vi "Left Click.vi"(7 "object refs":T2, 8 "error in (no error)":errorcluster, 9 "Coords":T1, 10 "Event data":variant, 11 "Data Grid in":refnum<class "Data Grid.lvclass">) -> (0 "error out":errorcluster, 2 "Discard?":bool, 3 "Data Grid out":refnum<class "Data Grid.lvclass">)   [LabVIEW 2013, in "Table Manager.lvlib" / "Data Grid.lvclass"]
uses:
  Data Grid.lvclass
  Table Manager/object ref.ctl
  <vilib>/NI/Tag Bus Data Framework/Configuration Editor/Classes/Engine Parent/Engine Parent Editor Node.lvclass
  <vilib>/NI/Tag Bus Data Framework/Configuration Editor/Classes/Module editor node/module editor node.lvclass
  <vilib>/Utility/miscctls.llb/LVPoint32TypeDef.ctl
  <vilib>/LabVIEW DataGridView/source/Events/Abstract EVENT/Abstract EVENT.lvclass
  Data Grid.lvclass/Data Grid.ctl
  Table Manager/Table Manager.lvclass/Table Manager.ctl
  Line/Line.lvclass/Line.ctl
  Column/Column.lvclass/Column.ctl
  Column/Column.lvclass
  Table Manager/Read ATM.vi
  Table Manager/Read Line.vi
  Table Manager/Read Top VI.vi
  Line/Read Columns.vi
  Line/Write Columns.vi
  Table Manager/Write Line.vi
  <vilib>/NI/Tag Bus Data Framework/Configuration Editor/Classes/Module editor node/Read Module Configuration.vi
  Line/Line.lvclass
  <vilib>/NI/Tag Bus Module Framework/module configuration/TBM module configuration.lvclass
  <vilib>/LabVIEW DataGridView/source/Events/CellClick/CellClick.lvclass
  <vilib>/NI/Tag Bus/tag/tag descriptor.lvclass
  Table Manager.lvlib
  <vilib>/LabVIEW DataGridView/source/DataGridView/DataGridView.lvclass
  Table Manager/Table Manager.lvclass
  Mapping Column/Mapping Column.lvclass
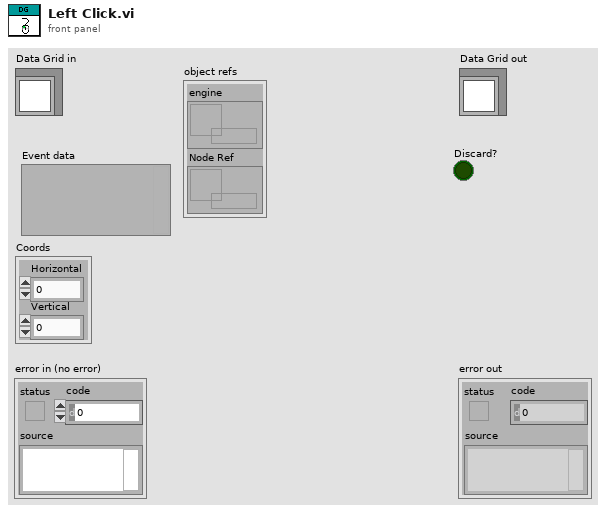
[diagram p1: front panel]
types:
  T1 = typedef "LVPoint32TypeDef.ctl" = cluster{"Horizontal":i32, "Vertical":i32}
  T2 = typedef "Table Manager.lvlib/Table Manager.lvclass/object ref.ctl" = cluster{"engine":refnum<data-value>, "Node Ref":refnum<data-value>}
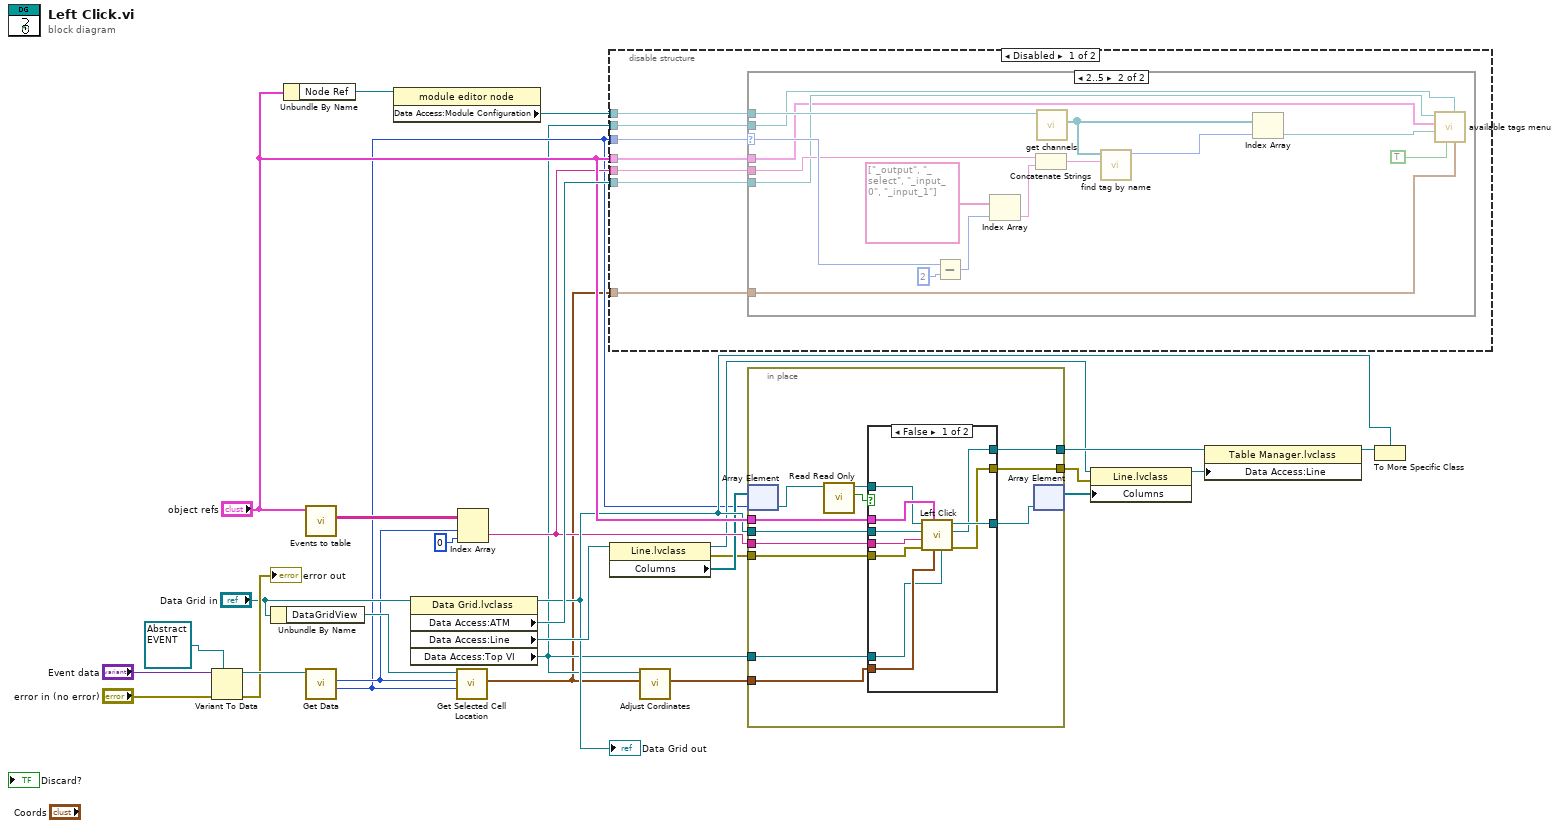
[diagram p0: block diagram]
diagram:
  n1 = Variant To Data(error in="error in (no error)", type=refnum<class "Abstract EVENT.lvclass"> refnum ("DataGrid.lvlib:Abstract EVENT.lvclass"), Variant="Event data") -> (data=w23:refnum<class "Abstract EVENT.lvclass">, error out=→"error out":errorcluster)
  n2 = Unbundle By Name("Data Grid in") -> ("DataGridView"=w22:refnum<class "DataGridView.lvclass">)
  n3 = Unbundle By Name("object refs") -> ("Node Ref"=w27:refnum<data-value>)
  n4 = call "Events to table.vi"("object ref in"="object refs") -> ("table"=w26:string[][])  [unwired: 8 in, 2 out]
  n5 = call <vilib>:"Get Data.vi"("DataGrid.lvlib:Abstract EVENT.lvclass"=w23) -> ("column"=w4:i32, "row"=w17:i32)  [unwired: 8 in, 1 out]
  n6 = property class="module editor node"(reference=w27) -> ("Data Access:Module Configuration"=w28:refnum<class "TBM module configuration.lvclass">)  [unwired: 1 in, 2 out]
  n7 = property class="Data Grid.lvclass"(reference="Data Grid in") -> (reference out=w14:refnum<class "Data Grid.lvclass">, "Data Access:ATM"=w18:refnum<user-event>, "Data Access:Line"=w16:refnum<class "Line.lvclass">, "Data Access:Top VI"=w3:refnum<vi>)  [unwired: 1 in, 1 out]
  "Data Grid out" <- w14
  n8 = call <vilib>:"Get Selected Cell Location.vi"("column"=w4, "row"=w17, "DataGridView in"=w22) -> ("Coords"=w2:T1)  [unwired: 7 in, 1 out]
  n9 = Index Array(array=w26, index (row)=w17, index (col)=0 ("disabled index (col)")) -> (element=w10:string)
  n10 = disable-structure shown="Disabled" {
    disable-tunnel: w2 -> [w36 _]
    disable-tunnel: w10 -> [w35 _]
    disable-tunnel: w28 -> [w34 _]
    disable-tunnel: w18 -> [w33 _]
    disable-tunnel: w4 -> [w32 _]
    disable-tunnel: w3 -> [w31 _]
    disable-tunnel: "object refs" -> [w30 _]
    frame Disabled {
      n11 = case shown="2..5" w32 {
        selector: w32 -> [_ w49]
        tunnel: w35 -> [_ w45]
        tunnel: w36 -> [_ w39]
        tunnel: w34 -> [_ w41]
        tunnel: w33 -> [_ w40]
        tunnel: w30 -> [_ w38]
        tunnel: w31 -> [_ w37]
        frame 0, Default {
        }
        frame 2..5 {
          n12 = Subtract(x=w49, y=2) -> (x-y=w48:i32)
          n13 = Index Array(array=string[] ["_output", "_select", "_input_0", "_input_1"], index=w48) -> (element=w44:string)
          n14 = Concatenate Strings(w45, w44) -> (w46:string)
          n15 = call-dynamic "get channels.vi"("module configuration in"=w41) -> ("channels"=w42:refnum<class "TBM channel.lvclass">[])  [unwired: 9 in, 1 out]
          n16 = call <vilib>:"find tag by name.vi"("name"=w46, "tags in"=w42) -> ("index"=w52:i32)  [unwired: 9 in]
          n17 = Index Array(array=w42, index=w52) -> (element=w51:refnum<class "TBM channel.lvclass">)
          n18 = call "available tags menu.vi"("Point32"=w39, "parent vi reference"=w37, "Screen"=TRUE, "channel to map to"=w51, "object ref"=w38, "ATM"=w40) -> ()  [unwired: 5 in, 1 out]
        }
      }
    }
    frame Enabled {
    }
  }
  n19 = property class="Line.lvclass"(reference=w16) -> (reference out=w7:refnum<class "Line.lvclass">, error out=w6:errorcluster, "Columns"=w9:refnum<class "Column.lvclass">[])  [unwired: 1 in]
  n20 = call "Adjust Cordinates.vi"("Point32"=w2, "VI in"=w3) -> ("Coords out"=w1:T1)  [unwired: 8 in, 1 out]
  n21 = in-place {
    in-place-border: "object refs" -> [w63]
    in-place-border: w14 -> [w62]
    in-place-border: [w61] -> w13
    in-place-border: w1 -> [w60]
    in-place-border: w10 -> [w59]
    in-place-border: w6 -> [w55]
    in-place-border: [w54] -> w5
    in-place-border: w3 -> [w53]
    n22 = in-place-array #1(w9, w4) -> (w58:refnum<class "Column.lvclass">)
    n23 = call "Read Read Only.vi"("Column in"=w58) -> ("Read Only"=w56:bool, "Column out"=w57:refnum<class "Column.lvclass">)  [unwired: 8 in, 1 out]
    n24 = case shown="False" w56 {
      tunnel: [w74 w77] -> w64
      tunnel: w63 -> [w73 _]
      tunnel: w62 -> [w72 w76]
      tunnel: [w71 w76] -> w61
      tunnel: w60 -> [w70 _]
      tunnel: w59 -> [w69 _]
      tunnel: w57 -> [w68 w77]
      tunnel: w55 -> [w67 w75]
      tunnel: [w66 w75] -> w54
      tunnel: w53 -> [w65 _]
      frame False {
        n25 = call-dynamic "Left Click.vi"("Top  VI"=w65, "Coords"=w70, "object refs"=w73, "error in (no error)"=w67, "line name"=w69, "Table Manager in"=w72, "column in"=w68) -> ("error out"=w66:errorcluster, "Table Manager out"=w71:refnum<class "Table Manager.lvclass">, "column out"=w74:refnum<class "Column.lvclass">)  [unwired: 1 in, 1 out]
      }
      frame True {
      }
    }
    n26 = in-place-array #1(w64) -> (w8:refnum<class "Column.lvclass">[])  [unwired: 1 out]
  }
  n27 = property class="Line.lvclass"(reference=w7, error in=w5, "Columns"=w8) -> (reference out=w12:refnum<class "Line.lvclass">)  [unwired: 1 out]
  n28 = property class="Table Manager.lvclass"(reference=w13, "Data Access:Line"=w12) -> (reference out=w11:refnum<class "Table Manager.lvclass">)  [unwired: 1 in, 1 out]
  n29 = To More Specific Class(target class=w14, reference=w11) -> ()  [unwired: 1 in, 2 out]
